vi "Transmit - Generic.vi"() -> ()   [LabVIEW 2020]
uses:
  <instrlib>/AIM GmbH/_AIM 664/_controls/queue_data_full.ctl
  <instrlib>/AIM GmbH/_AIM 664/_controls/queue_header_generic.ctl
  <instrlib>/AIM GmbH/_AIM 664/_polimorphicInstances/session/CreateSession(Tx-Generic).vi
  <instrlib>/AIM GmbH/_AIM 664/_polimorphicInstances/control/Start (Tx).vi
  <instrlib>/AIM GmbH/_AIM 664/_polimorphicInstances/control/Stop (Tx).vi
  <instrlib>/AIM GmbH/_AIM 664/_polimorphicInstances/session/CleanupSession (Port).vi
  <instrlib>/AIM GmbH/_AIM 664/AIM664LV.lvlib
panel:
  in  "Period mS":u32=200
  out "TxStatus":T1
  out "TxQueueStatus":T2 {"QueueStatus" items=["FDX_QUE_EMPTY", "FDX_QUE_FILLED", "FDX_QUE_FULL", "FDX_QUE_SENT", "FDX_QUE_CYCL_RUN", "FDX_QUE_CYCL_SENT"]}
  in  "HeaderInfo":T3={"InterFrameGap"=0, "PacketGroupWaitTime"=10000, "PayloadBufferMode"=0, "PayloadGenerationMode"=0, "PreambleCount"=7, "Skew"=0, "NetSelect"=4, "FrameStartMode"=1, "PhysErrorInjection"=0, "SequenceNumberInit"=65535, "SequenceNumberOffset"=65535} {"NetSelect" items=["FDX_TX_FRAME_DLY_A"=0, "FDX_TX_FRAME_DLY_B"=1, "FDX_TX_FRAME_BOTH "=3, "FDX_TX_FRAME_ONLY_A"=4, "FDX_TX_FRAME_ONLY_B "=5]; "FrameStartMode" items=["FDX_TX_FRAME_START_IFG", "FDX_TX_FRAME_START_PGWT", "FDX_TX_FRAME_START_TRG"]; "PhysErrorInjection" items=["FDX_TX_FRAME_ERR_OFF"=0, "FDX_TX_FRAME_ERR_CRC"=1, "FDX_TX_FRAME_ERR_ALI"=2, "FDX_TX_FRAME_ERR_PRE"=4, "FDX_TX_FRAME_ERR_PHY"=8]; "SequenceNumberInit" items=["FDX_TX_FRAME_SEQ_INIT_AUTO"=65535]; "SequenceNumberOffset" items=["FDX_TX_FRAME_SEQ_OFFS_AUTO "=65535]; "PayloadGenerationMode" items=["FDX_TX_FRAME_PGM_USER"=0, "FDX_TX_FRAME_PGM_IP_PART"=1, "FDX_TX_FRAME_PGM_IP_FULL"=2, "FDX_TX_FRAME_PGM_IP_PART_TT"=10, "FDX_TX_FRAME_PGM_IP_FULL_TT"=20]; "PayloadBufferMode" items=["FDX_TX_FRAME_PBM_STD", "FDX_TX_FRAME_PBM_MAC", "FDX_TX_FRAME_PBM_UDP"]}
  out "TxQueueInfo":cluster{"QueueBaseAddr":u32, "QueueSizeOut":u32}
  in  "VL Id":u16=60
  in  "UDPdstPort":u16=1
  in  "UDPsrcPort":u16=1
  in  "Frame Configuration":T4={"domainID"=1, "sideID"=1, "locationID"=1, "interfaceID"=1, "partitionID"=1} {"interfaceID" format="%.0b"}
  in  "QueueSizeIn":u32
  in  "Frame payload size (bytes)":i32=100
  out "Curent Irig Time":T5
  out "Data":u8[](array[numeric])=[10] format="%.0x"
  out "PortInitOut":T6 {"PortConfig" items=["FDX_SINGLE", "FDX_REDUNDANT"]}
  in  "port":u32
  in  "board":u32
  out "error out":errorcluster
  in  "stop":bool
  out "current time":timestamp
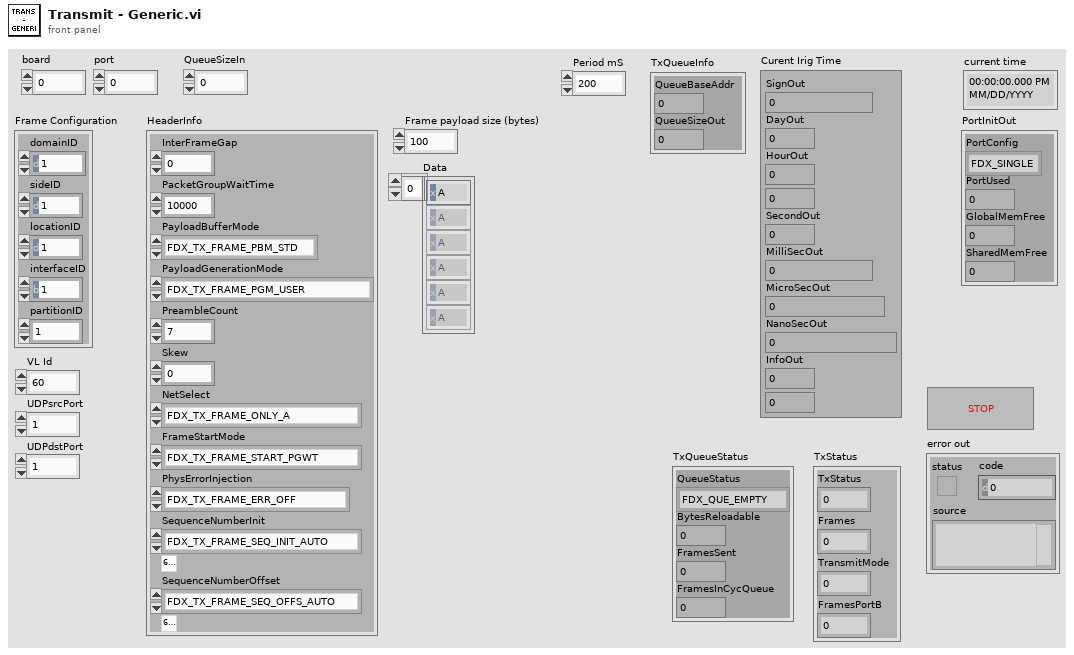
[diagram p1: front panel]
types:
  T1 = cluster{"TxStatus":u32, "Frames":u32, "TransmitMode":u32, "FramesPortB":u32}
  T2 = cluster{"QueueStatus":i32, "BytesReloadable":u32, "FramesSent":u32, "FramesInCycQueue":u32}
  T3 = typedef "AIM664LV.lvlib/queue_header_generic.ctl" = cluster{"InterFrameGap":u32, "PacketGroupWaitTime":u32, "PayloadBufferMode":u8, "PayloadGenerationMode":u8, "PreambleCount":u8, "Skew":u32, "NetSelect":u8, "FrameStartMode":u8, "PhysErrorInjection":u32, "SequenceNumberInit":u16, "SequenceNumberOffset":u16}
  T4 = typedef "AIM664LV.lvlib/queue_data_full.ctl" = cluster{"domainID":u8, "sideID":u8, "locationID":u8, "interfaceID":u8, "partitionID":u8}
  T5 = cluster{"SignOut":i32, "DayOut":u32, "HourOut":u32, "MinOut":u32, "SecondOut":u32, "MilliSecOut":u32, "MicroSecOut":u32, "NanoSecOut":u32, "InfoOut":u32, "Mode":u32}
  T6 = cluster{"PortConfig":u32, "PortUsed":u32, "GlobalMemFree":u32, "SharedMemFree":u32}
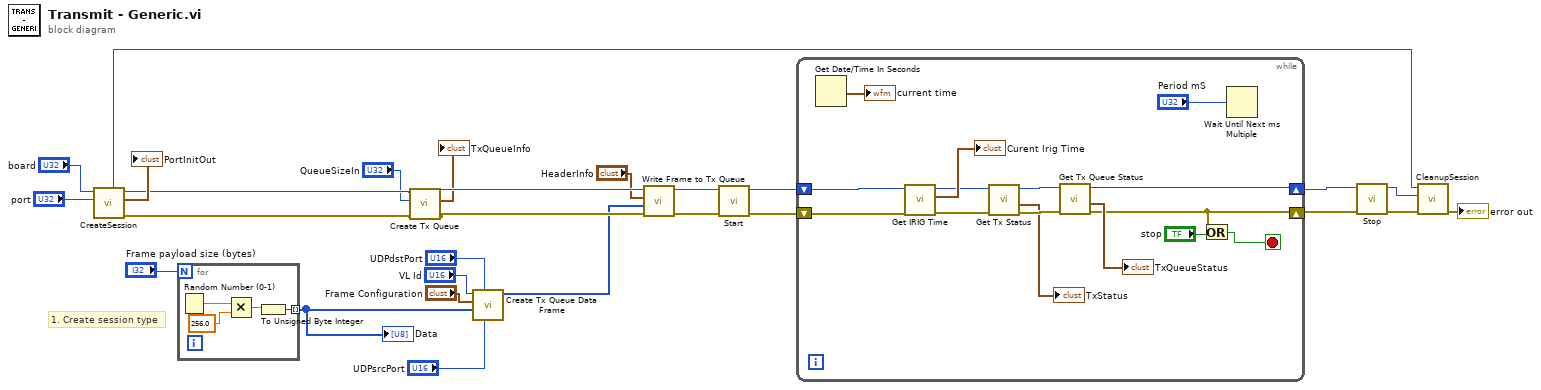
[diagram p0: block diagram]
diagram:
  # "1. Create session type"
  n1 = call-poly <instrlib>:"CreateSession.vi"("port"="port", "board"="board") -> ("error out"=w18:errorcluster, "PortInitOut"=→"PortInitOut":T6, "port handle out"=w19:u32, "InstrumentHandle_board out"=w3:u32)  [unwired: 5 in, 1 out]
  n2 = for {
    N: "Frame payload size (bytes)" -> [_]
    tunnel: [w28] -> w12 mode=indexing
    n3 = Random Number (0-1)() -> (number: 0 to 1=w31:dbl)
    n4 = Multiply(x=w31, y=256.0) -> (x*y=w29:dbl)
    n5 = To Unsigned Byte Integer(number=w29) -> (unsigned 8bit integer=w28:u8)
  }
  "Data" <- w12
  n6 = call <instrlib>:"Create Tx Queue.vi"("error in (no error)"=w18, "QueueSizeIn"="QueueSizeIn", "InstrumentHandle_port in"=w19) -> ("error out"=w9:errorcluster, "TxQueueInfo"=→"TxQueueInfo":cluster{"QueueBaseAddr":u32, "QueueSizeOut":u32}, "InstrumentHandle_port out"=w11:u32)  [unwired: 6 in]
  n7 = call <instrlib>:"Create Tx Queue Data Frame.vi"("UDPsrcPort"="UDPsrcPort", "UDPdstPort"="UDPdstPort", "Payload"=w12, "afdx configuration"="Frame Configuration", "VL Id"="VL Id") -> ("Frame"=w8:u8[])  [unwired: 6 in]
  n8 = call <instrlib>:"Write Frame to Tx Queue.vi"("error in (no error)"=w9, "Frame in"=w8, "HeaderInfo"="HeaderInfo", "InstrumentHandle_port in"=w11) -> ("error out"=w7:errorcluster, "InstrumentHandle_port out"=w6:u32)  [unwired: 6 in]
  n9 = call-poly <instrlib>:"Start.vi"("error in (no error)"=w7, "InstrumentHandle_port in"=w6) -> ("error out"=w1:errorcluster, "InstrumentHandle_port out"=w27:u32)  [unwired: 8 in]
  n10 = while {
    shift-right: [w40] -> w26
    shift-left: w27 -> [w45]
    shift-right: [w34] -> w2
    shift-left: w1 -> [w33]
    stop <- w35 stop-if-true
    n11 = Get Date/Time In Seconds() -> (seconds since 1Jan1904=→"current time":timestamp)
    n12 = call <instrlib>:"Get IRIG Time.vi"("error in (no error)"=w33, "InstrumentHandle_board in"=w45) -> ("error out"=w39:errorcluster, "Curent Irig Time"=→"Curent Irig Time":T5, "InstrumentHandle_board out"=w43:u32)  [unwired: 7 in]
    n13 = call <instrlib>:"Get Tx Status.vi"("error in (no error)"=w39, "InstrumentHandle_port in"=w43) -> ("error out"=w41:errorcluster, "TxStatus"=→"TxStatus":T1, "InstrumentHandle_port out"=w42:u32)  [unwired: 7 in]
    n14 = call <instrlib>:"Get Tx Queue Status.vi"("error in (no error)"=w41, "InstrumentHandle in"=w42) -> ("error out"=w34:errorcluster, "TxQueueStatus"=→"TxQueueStatus":T2, "InstrumentHandle out"=w40:u32)  [unwired: 7 in]
    n15 = Or(x=w34, y="stop") -> (x .or. y?=w35:bool)
    n16 = Wait Until Next ms Multiple(millisecond multiple="Period mS") -> ()  [unwired: 1 out]
  }
  n17 = call-poly <instrlib>:"Stop.vi"("error in (no error)"=w2, "InstrumentHandle_port in"=w26) -> ("error out"=w21:errorcluster, "InstrumentHandle_port out"=w4:u32)  [unwired: 8 in]
  n18 = call-poly <instrlib>:"CleanupSession.vi"("error in (no error)"=w21, "InstrumentHandle_port in"=w4, "InstrumentHandle_board in"=w3) -> ("error out"=→"error out":errorcluster)  [unwired: 8 in]
